vi "XYcordenadas_a_stringINT.vi"(8 "fin de cadena":string=" S", 10 "y":i32, 11 "x":i32) -> (2 "String":string, 5 "ok":bool)   [LabVIEW 2017]
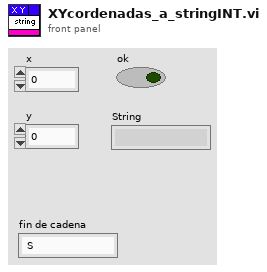
[diagram p1: front panel]
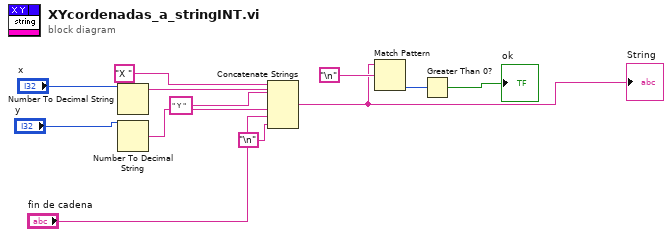
[diagram p0: block diagram]
diagram:
  n1 = Number To Decimal String(number="x") -> (decimal integer string=w4:string)  [unwired: 1 in]
  n2 = Number To Decimal String(number="y") -> (decimal integer string=w6:string)  [unwired: 1 in]
  n3 = Concatenate Strings("X " ("string"), w4, " Y " ("string"), w6, "fin de cadena", "\n") -> (w9:string)
  "String" <- w9
  n4 = Match Pattern(string=w9, regular expression="\n") -> (offset past match=w11:i32)  [unwired: 1 in, 3 out]
  n5 = Greater Than 0?(x=w11) -> (x > 0?=→"ok":bool)
